vi "SysParamsSave.vi"(7 "Path":path, 8 "error in (no error)":errorcluster, 11 "AirSAS Controls":T1={"Receive Duration"=0.0, "I/O"={"DAQmx Device"="Dev1", "AO Range"=0.0, "AI Range"=0.0, "DAQ Group Delay"=0.0, "Fs"=0.0}, "Hardware"={"Centerpos"=[0.0, 0.0, 0.0], "TXpos"=[0.0, 0.0, 0.0], "RX1pos"=[0.0, 0.0, 0.0], "RX2pos"=[0.0, 0.0, 0.0], "Angle"=0.0, "Height"=0.0}, "Waveform"={"LFM Parameters"={"Duration"=1.0, "Fstart (Hz)"=1000.0, "Fstop (Hz)"=10000.0, "Out. Amplitude (Vpk)"=1.0, "Window %"=10.0}, "Transmit Waveform"={"t0"=timestamp(0 s since 1904-01-01), "dt"=1.0, "Y"=[]}}, "LINX Resource"={"IO"=enum."Remote", "Interface"=enum."Serial", "LINX Device Config"={"Interface"=enum."Serial", "COM Port"="COM13", "TCP Configuration"={"IP Address"="", "Port"=0}, "Device Family"=1, "Device ID"=1, "Device Name"="myRIO-1900", "TCP Ref"=refnum, "Channels"={"DI"=[0, 1, 2, 3, 4, 5, 6, 7, 8, 9, 10, 11, 12, 13, 14, 15, 16, 17, 18, 19, 20, 21, 22, 23, 24, 25, 26, 27, 28, 29, 30, 31, 32, 33, 34, 35, 36, 37, 38, 39, 40, 41, 42, 43, 44, 45, 46], "DO"=[0, 1, 2, 3, 4, 5, 6, 7, 8, 9, 10, 11, 12, 13, 14, 15, 16, 17, 18, 19, 20, 21, 22, 23, 24, 25, 26, 27, 28, 29, 30, 31, 32, 33, 34, 35, 36, 37, 38, 39, 40, 41, 42, 43, 44, 45, 46], "AI"=[0, 1, 2, 3, 4, 5, 6, 7, 8, 9, 10, 11], "AO"=[], "PWM"=[3, 5, 6, 9, 10], "QE"=[], "UART"=[0, 1], "I2C 2"=[0], "SPI"=[0], "CAN"=[], "Servo"=[], "AI Ref (V)"=0.0, "AI Resolution (Bits)"=0, "AO Ref (V)"=0.0, "AO Resolution (Bits)"=0}}}, "Port"=3000.0} {"Waveform"."LFM Parameters"."Window %" format="%.2g"; "Waveform"."LFM Parameters"."Out. Amplitude (Vpk)" format="%0.2f"; "Waveform"."LFM Parameters"."Fstop (Hz)" format="%^.3e"; "Waveform"."LFM Parameters"."Fstart (Hz)" format="%^.3e"; "Waveform"."LFM Parameters"."Duration" format="%.3f"}) -> (0 "error out":errorcluster)   [LabVIEW 2021]
uses:
  controls/Air SAS Controls.ctl
  <vilib>/MakerHub/LINX/Private/Type Defs/LINX Ref.ctl
  <vilib>/MakerHub/LINX/Private/Type Defs/Platform.ctl
  <vilib>/MakerHub/LINX/Private/Type Defs/Interface.ctl
  <vilib>/MakerHub/LINX/Private/Device/Type Defs/LINX Device Config.ctl
  <vilib>/MakerHub/LINX/Private/Device/Type Defs/TCP Config.ctl
  <vilib>/MakerHub/LINX/Private/Device/Type Defs/Channels.ctl
  <vilib>/Utility/file.llb/Write Delimited Spreadsheet (string).vi
  <vilib>/MakerHub/LINX/LMH-LINX.lvlib
  <vilib>/MakerHub/LINX/Private/Device/Device.lvlib
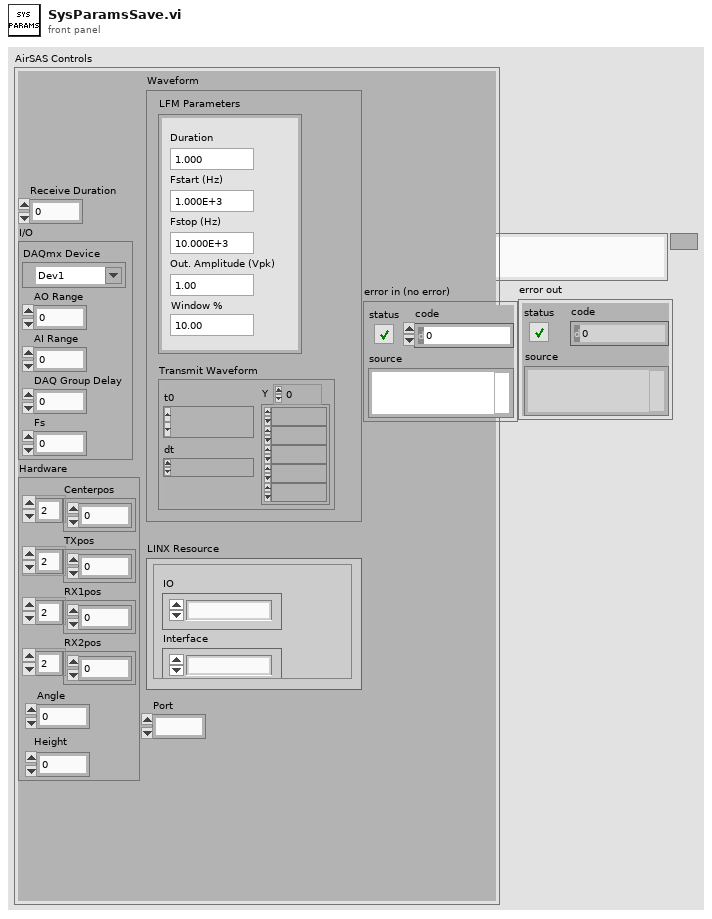
[diagram p1: front panel]
types:
  T1 = typedef "Air SAS Controls.ctl" = cluster{"Receive Duration":dbl, "I/O":cluster{"DAQmx Device":tag, "AO Range":dbl, "AI Range":dbl, "DAQ Group Delay":dbl, "Fs":dbl}, "Hardware":cluster{"Centerpos":dbl[], "TXpos":dbl[], "RX1pos":dbl[], "RX2pos":dbl[], "Angle":dbl, "Height":dbl}, "Waveform":cluster{"LFM Parameters":cluster{"Duration":dbl, "Fstart (Hz)":dbl, "Fstop (Hz)":dbl, "Out. Amplitude (Vpk)":dbl, "Window %":dbl}, "Transmit Waveform":waveform(dbl)}, "LINX Resource":T2, "Port":dbl}
  T2 = typedef "LMH-LINX.lvlib/LINX Ref.ctl" = cluster{"IO":T3, "Interface":T4, "LINX Device Config":T5}
  T3 = typedef "LMH-LINX.lvlib/Platform.ctl" = enum16{"Remote", "Local"}
  T4 = typedef "LMH-LINX.lvlib/Interface.ctl" = enum16{"Serial", "TCP"}
  T5 = typedef "LMH-LINX.lvlib/Device.lvlib/LINX Device Config.ctl" = cluster{"Interface":T4, "COM Port":refnum<visa-resource-name>, "TCP Configuration":T6, "Device Family":u8, "Device ID":u8, "Device Name":string, "TCP Ref":refnum<k5>, "Channels":T7}
  T6 = typedef "LMH-LINX.lvlib/Device.lvlib/TCP Config.ctl" = cluster{"IP Address":string, "Port":u16}
  T7 = typedef "LMH-LINX.lvlib/Channels.ctl" = cluster{"DI":u8[], "DO":u8[], "AI":u8[], "AO":u8[], "PWM":u8[], "QE":u8[], "UART":u8[], "I2C 2":u8[], "SPI":u8[], "CAN":u8[], "Servo":u8[], "AI Ref (V)":dbl, "AI Resolution (Bits)":u8, "AO Ref (V)":dbl, "AO Resolution (Bits)":u8}
  T8 = cluster{"DAQmx Device":tag, "AO Range":dbl, "AI Range":dbl, "DAQ Group Delay":dbl, "Fs":dbl}
  T9 = cluster{"Centerpos":dbl[], "TXpos":dbl[], "RX1pos":dbl[], "RX2pos":dbl[], "Angle":dbl, "Height":dbl}
  T10 = cluster{"Duration":dbl, "Fstart (Hz)":dbl, "Fstop (Hz)":dbl, "Out. Amplitude (Vpk)":dbl, "Window %":dbl}
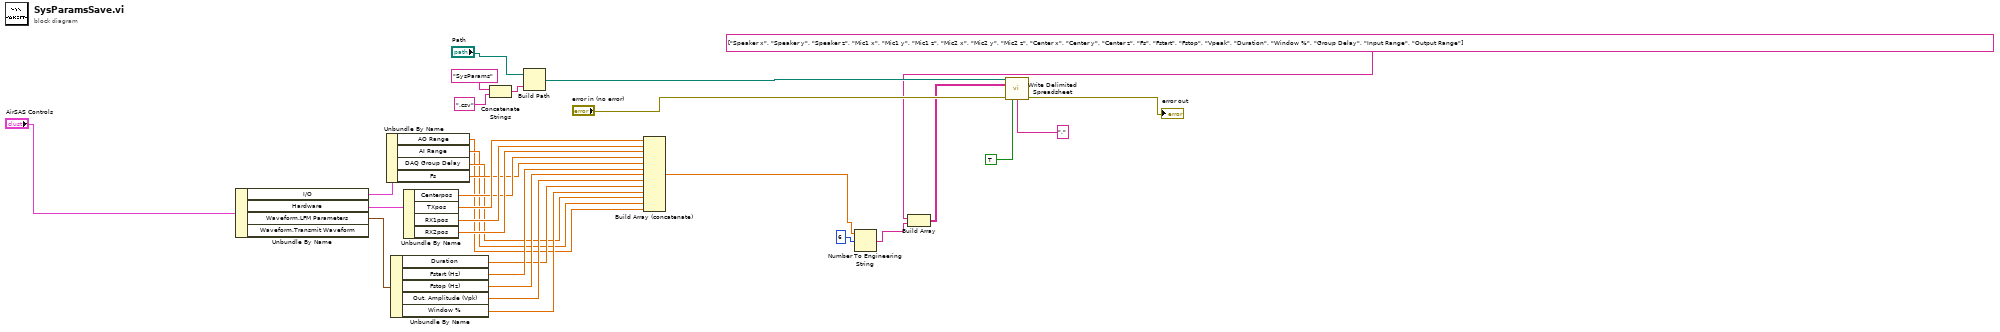
[diagram p0: block diagram]
diagram:
  n1 = Unbundle By Name("AirSAS Controls") -> ("I/O"=w31:T8, "Hardware"=w30:T9, "Waveform.LFM Parameters"=w29:T10)  [unwired: 1 out]
  n2 = Unbundle By Name(w31) -> ("AO Range"=w11:dbl, "AI Range"=w12:dbl, "DAQ Group Delay"=w13:dbl, "Fs"=w19:dbl)
  n3 = Unbundle By Name(w29) -> ("Duration"=w15:dbl, "Fstart (Hz)"=w18:dbl, "Fstop (Hz)"=w17:dbl, "Out. Amplitude (Vpk)"=w16:dbl, "Window %"=w14:dbl)
  n4 = Unbundle By Name(w30) -> ("Centerpos"=w20:dbl[], "TXpos"=w23:dbl[], "RX1pos"=w22:dbl[], "RX2pos"=w21:dbl[])
  n5 = Concatenate Strings("SysParams" ("string"), ".csv") -> (w27:string)
  n6 = Build Path(base path="Path", name or relative path=w27) -> (appended path=w24:path)
  n7 = Build Array (concatenate)(w23, w22, w21, w20, w19, w18, w17, w16, w15, w14, w13, w12, w11) -> (w3:dbl[])
  n8 = Number To Engineering String(3:i16 6 ("width (-)"), 4:w3) -> (0:w2:string[])  [unwired: 2 in]
  n9 = Build Array(string[] ["Speaker x", "Speaker y", "Speaker z", "Mic1 x", "Mic1 y", "Mic1 z", "Mic2 x", "Mic2 y", "Mic2 z", "Center x", "Center y", "Center z", "Fs", "Fstart", "Fstop", "Vpeak", "Duration", "Window %", "Group Delay", "Input Range", "Output Range"], w2) -> (w5:string[][])
  n10 = call-poly <vilib>:"Write Delimited Spreadsheet.vi"("file path (dialog if empty)"=w24, "2D data"=w5, "error in (no error)"="error in (no error)", "transpose? (no:F)"=TRUE, "delimiter (\\t)"="," ("delimiter (\\t)")) -> ("error out"=→"error out":errorcluster)  [unwired: 9 in, 1 out]
